vi "SRS Lockin CleanUp Data.vi"(8 "error in (no error)":errorcluster, 11 "VISA resource name":refnum<visa-resource-name>="GPIB0::10::INSTR") -> (0 "error out":errorcluster, 3 "VISA resource name out":refnum<visa-resource-name>="GPIB0::10::INSTR")   [LabVIEW 2015]
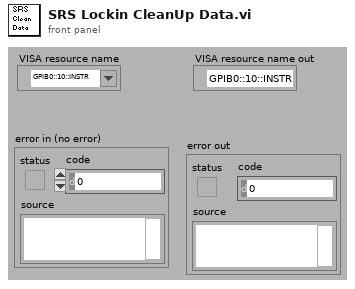
[diagram p1: front panel]
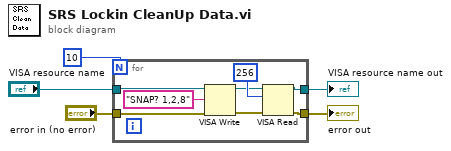
[diagram p0: block diagram]
diagram:
  n1 = for {
    N: 10 -> [_]
    tunnel: "VISA resource name" -> [w9]
    tunnel: "error in (no error)" -> [w6]
    tunnel: [w8] -> w2
    tunnel: [w7] -> w1
    n2 = VISA Write(VISA resource name=w9, write buffer="SNAP? 1,2,8", error in (no error)=w6) -> (VISA resource name out=w12:refnum<visa-resource-name>, error out=w11:errorcluster)  [unwired: 1 out]
    n3 = VISA Read(VISA resource name=w12, byte count=u32 256, error in (no error)=w11) -> (VISA resource name out=w8:refnum<visa-resource-name>, error out=w7:errorcluster)  [unwired: 2 out]
  }
  "VISA resource name out" <- w2
  "error out" <- w1
